vi "Close Starter Kit.vi"(8 "error in (no error)":errorcluster, 11 "starter kit host in":refnum<class "NI_Robotics_Starter Kit Host_FPGA_2.0.lvclass">) -> (0 "error out":errorcluster)   [LabVIEW 2017, in "NI_Robotics_Starter Kit Host_FPGA_2.0.lvclass"]
uses:
  <vilib>/robotics/Starter Kit/2.0/FPGA Host Interface/NI_Robotics_Starter Kit Host_FPGA_2.0.lvclass
  <vilib>/robotics/Starter Kit/2.0/FPGA Host Interface/NI_Robotics_Starter Kit Host_FPGA_2.0.lvclass/NI_Robotics_Starter Kit Host_FPGA_2.0.ctl
  <vilib>/FPGAPlugInAG/Dynamic/niLvFpga_Close_Dynamic.vi
  <vilib>/rvi/errors/niLvFpgaAdjustHostInterfaceError.vi
  <vilib>/Utility/error.llb/Error Cluster From Error Code.vi
  <vilib>/rvi/interface/nirviCloseFPGA/nirviCloseFPGA.xnode
  <vilib>/robotics/Starter Kit/2.0/FPGA Host Interface/FPGA Refnum.ctl
  <vilib>/rvi/interface/nirviReadWriteControl/nirviReadWriteControl.xnode
  NiFpgaLv.dll
  <vilib>/rvi/interface/Simulation/niFpgaSimulationCallBeginRW.vi
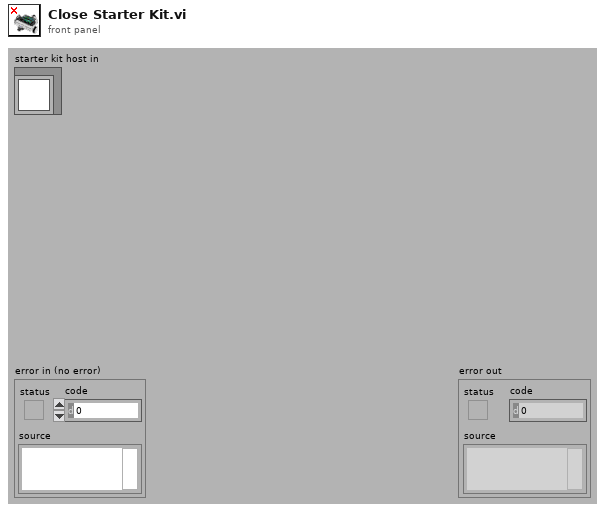
[diagram p1: front panel]
types:
  T1 = typedef "NI_Robotics_Starter Kit Host_FPGA_2.0.lvclass/FPGA Refnum.ctl" = refnum<k20>
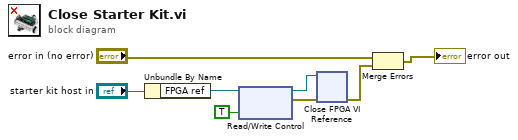
[diagram p0: block diagram]
diagram:
  n1 = Unbundle By Name("starter kit host in") -> ("FPGA ref"=w6:T1)
  n2 = xnode "Read/Write Control"("FPGA VI Reference In"=w6, "stop"=TRUE) -> ("FPGA VI Reference Out"=w7:T1, "error out"=w5:errorcluster)  [unwired: 1 in]
  n3 = xnode "Close FPGA VI Reference"("FPGA VI Reference In"=w7, "error in"=w5) -> ("error out"=w8:errorcluster)
  n4 = Merge Errors("error in (no error)", w8) -> (→"error out":errorcluster)
